vi "User Example - Python.vi"() -> ()   [LabVIEW 2019, in "xy_utilities.lvlib"]
uses:
  User.Python/User.Python.lvclass/User.Python.ctl
  User/User (single).vi
  User.Python/User.Python.lvclass
  C:/Users/patrick/Documents/GitHub/ciozi137/XY-Utilities/src/User/User.lvclass
  User/User.lvclass
  xy_utilities.lvlib
panel:
  out "error out":errorcluster
  in  "function name":string="NumpyMath"
  in  "operation":string
  out "XY-data out":cluster{"X-array":dbl[], "Y-array":dbl[]} {"Y-array" format="%.2p"; "X-array" format="%.2p"}
  # "XY_NumpyMath\nNumpyMath"
  # "Operations:\nadd: element-wise addition (x + y)\nmultiply: element-wise multiplication (x * y)\nnorm_x: L2 norm of x\nnorm_y: L2 norm of y\ndot: dot product of x and y (using matmul)"
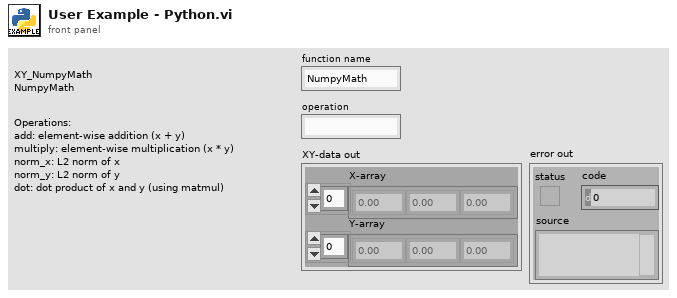
[diagram p1: front panel]
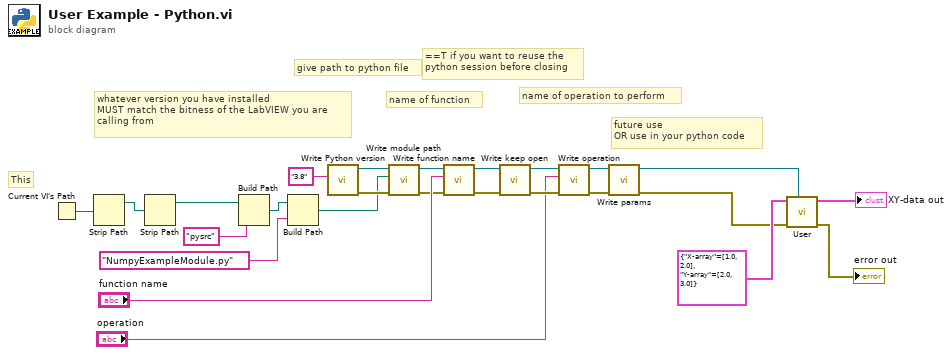
[diagram p0: block diagram]
diagram:
  # "future use\nOR use in your python code"
  # "name of operation to perform"
  # "==T if you want to reuse the\npython session before closing"
  # "name of function"
  # "give path to python file"
  # "This"
  # "whatever version you have installed\nMUST match the bitness of the LabVIEW you are\ncalling from"
  n1 = Current VI's Path() -> (path=w19:path)
  n2 = Strip Path(path=w19) -> (stripped path=w9:path)  [unwired: 1 out]
  n3 = Strip Path(path=w9) -> (stripped path=w8:path)  [unwired: 1 out]
  n4 = Build Path(base path=w8, name or relative path="pysrc") -> (appended path=w10:path)
  n5 = Build Path(base path=w10, name or relative path="NumpyExampleModule.py") -> (appended path=w18:path)
  n6 = call "Write Python version.vi"("Python version"="3.8") -> ("error out"=w21:errorcluster, "User.Python out"=w24:refnum<class "User.Python.lvclass">)  [unwired: 9 in]
  n7 = call "Write module path.vi"("error in (no error)"=w21, "module path"=w18, "User.Python in"=w24) -> ("error out"=w20:errorcluster, "User.Python out"=w23:refnum<class "User.Python.lvclass">)  [unwired: 7 in]
  n8 = call "Write function name.vi"("error in (no error)"=w20, "function name"="function name", "User.Python in"=w23) -> ("error out"=w15:errorcluster, "User.Python out"=w17:refnum<class "User.Python.lvclass">)  [unwired: 7 in]
  n9 = call "Write keep open.vi"("error in (no error)"=w15, "User.Python in"=w17) -> ("error out"=w14:errorcluster, "User.Python out"=w16:refnum<class "User.Python.lvclass">)  [unwired: 8 in]
  n10 = call "Write operation.vi"("error in (no error)"=w14, "operation"="operation", "User.Python in"=w16) -> ("error out"=w4:errorcluster, "User.Python out"=w3:refnum<class "User.Python.lvclass">)  [unwired: 7 in]
  n11 = call "Write params.vi"("error in (no error)"=w4, "User.Python in"=w3) -> ("error out"=w1:errorcluster, "User.Python out"=w2:refnum<class "User.Python.lvclass">)  [unwired: 8 in]
  n12 = call-poly "User.vi"("User.lvclass"=w2, "error in (no error)"=w1, "XY-data"=cluster{"X-array":dbl[], "Y-array":dbl[]} {"X-array"=[1.0, 2.0], "Y-array"=[2.0, 3.0]}) -> ("error out"=→"error out":errorcluster, "XY-data out"=→"XY-data out":cluster{"X-array":dbl[], "Y-array":dbl[]})  [unwired: 6 in, 1 out]
